vi "DraggingDresser.vi"() -> ()   [LabVIEW 2014]
panel:
  out "Force":dbl[](array[numeric])
  out "Angle for Minimum Force":i32 format="%.1f"
  in  "Coefficient of Kinetic Friction":dbl format="%.1f"
  out "Waveform Graph":dbl[](graph)
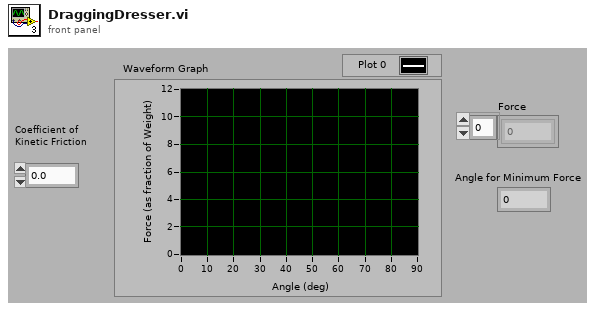
[diagram p1: front panel]
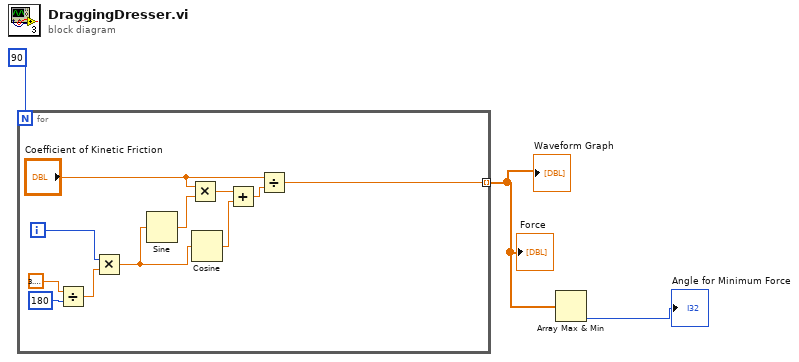
[diagram p0: block diagram]
diagram:
  n1 = for {
    N: 90 -> [_]
    tunnel: [w9] -> w2 mode=indexing
    i -> [w4]
    n2 = Divide(x=3.141592653589793, y=180) -> (x/y=w6:dbl)
    n3 = Multiply(x=w4, y=w6) -> (x*y=w5:dbl)
    n4 = Sine(x=w5) -> (sin(x)=w14:dbl)
    n5 = Multiply(x="Coefficient of Kinetic Friction", y=w14) -> (x*y=w12:dbl)
    n6 = Cosine(x=w5) -> (cos(x)=w13:dbl)
    n7 = Add(x=w12, y=w13) -> (x+y=w10:dbl)
    n8 = Divide(x="Coefficient of Kinetic Friction", y=w10) -> (x/y=w9:dbl)
  }
  "Waveform Graph" <- w2
  "Force" <- w2
  n9 = Array Max & Min(array=w2) -> (min index (indices)=→"Angle for Minimum Force":i32)  [unwired: 3 out]
